vi "Get Attribute without specifierRequirement.vi"() -> ()   [LabVIEW 2023]
uses:
  <vilib>/regexp/Match Regular Expression.xnode
panel:
  in  "specifierRequirement":string="SpecAnListStep"
  out "Attributes without specified specifierRequirement":string[](array[string])
  in  "Attributes xml path":path
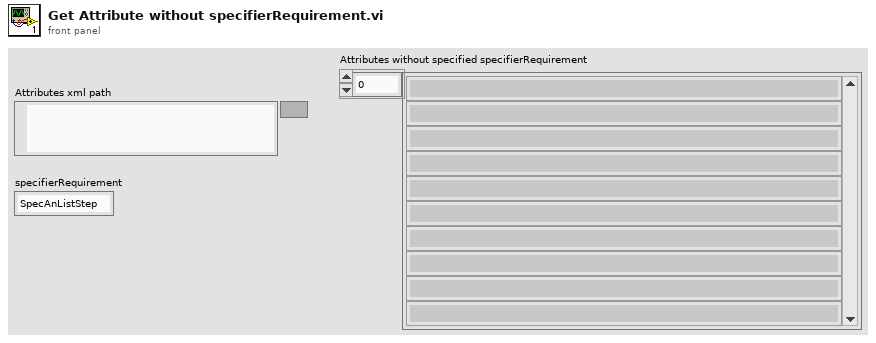
[diagram p1: front panel]
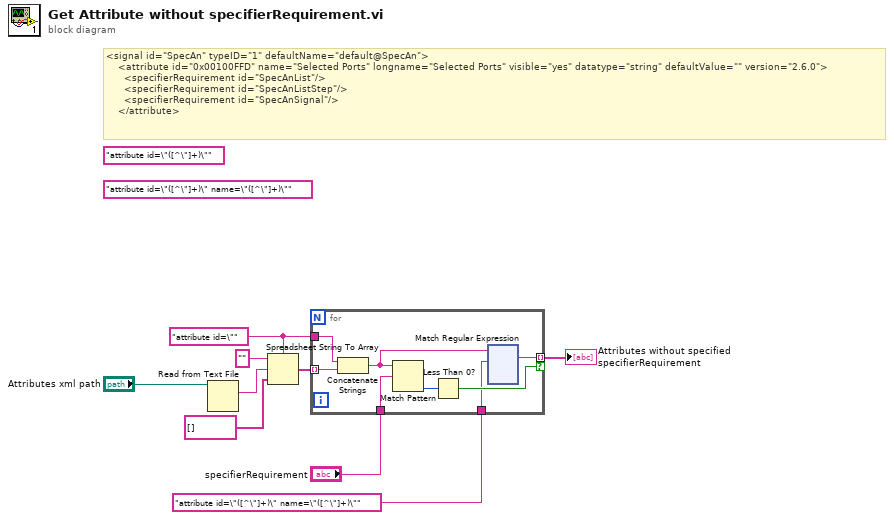
[diagram p0: block diagram]
diagram:
  w3 = "attribute id=\"" ("regular expression")
  (unwired) "attribute id=\"([^\"]+)\" name=\"([^\"]+)\"" ("regular expression")
  (unwired) "attribute id=\"([^\"]+)\"" ("regular expression")
  # "<signal id=\"SpecAn\" typeID=\"1\" defaultName=\"default@SpecAn\">\n    <attribute id=\"0x00100FFD\" name=\"Selected Ports\" longname=\"Selected Ports\" visible=\"yes\" datatype=\"string\" defaultValue=\"\" version=\"2.6.0\">\n      <specifierRequirement id=\"SpecAnList\"/>\n      <specifierRequirement id=\"SpecAnListStep\"/>\n      <specifierRequirement id=\"SpecAnSignal\"/>\n    </attribute>"
  n1 = Read from Text File(file (use dialog)="Attributes xml path") -> (text=w4:string)  [unwired: 3 in, 3 out]
  n2 = Spreadsheet String To Array(delimiter (Tab)=w3, format string="", spreadsheet string=w4, array type (2D Dbl)=string[] [] ("format string")) -> (array=w5:string[])
  n3 = for {
    tunnel: w5 -> [w16] mode=indexing
    tunnel: [w12] -> w8 mode=indexing if=w15
    tunnel: w3 -> [w13]
    tunnel: "specifierRequirement" -> [w11]
    tunnel: "attribute id=\"([^\"]+)\" name=\"([^\"]+)\"" ("regular expression") -> [w10]
    n4 = Concatenate Strings(w13, w16) -> (w14:string)
    n5 = Match Pattern(string=w14, regular expression=w11) -> (offset past match=w17:i32)  [unwired: 1 in, 3 out]
    n6 = Less Than 0?(x=w17) -> (x < 0?=w15:bool)
    n7 = xnode "Match Regular Expression"("input string"=w14, "regular expression"=w10) -> ("whole match"=w12:string)  [unwired: 4 in, 4 out]
  }
  "Attributes without specified specifierRequirement" <- w8
